vi "BMark_User Visible Strings.vi"() -> ()   [LabVIEW 2013]
panel:
  in  "Switch App Instance":string="LabVIEW cannot locate the specified application instance. "
  in  "Cannot Highlight (missing)":string="The reference for this label is no longer valid."
  in  "Cannot Highlight (lock)":string="Front panel objects in a locked VI (or a VI without a block diagram) cannot be highlighted."
  in  "Cannot Highlight (VI moved)":string="The VI you are trying to open was moved, deleted, or renamed."
  in  "Cannot Highlight (pwd)":string="Labels in a password-protected VI cannot be highlighted if the password is not in the cache."
  in  "Cannot Highlight (run)":string="You cannot highlight labels in a running VI (or a subVI of a running VI)."
  in  "Populating list":string="Populating list... Please wait"
  in  "More Information":string="More Information"
  in  "no bookmarks found":string="No bookmarks found."
  in  "Bookmarks":string="Bookmarks"
  in  "VIs":string="VIs"
  in  "Main application instance":string="Main Application Instance"
  in  "unknown message error":string="The invalid message string \"%s\" was received in the Message Handling Loop."
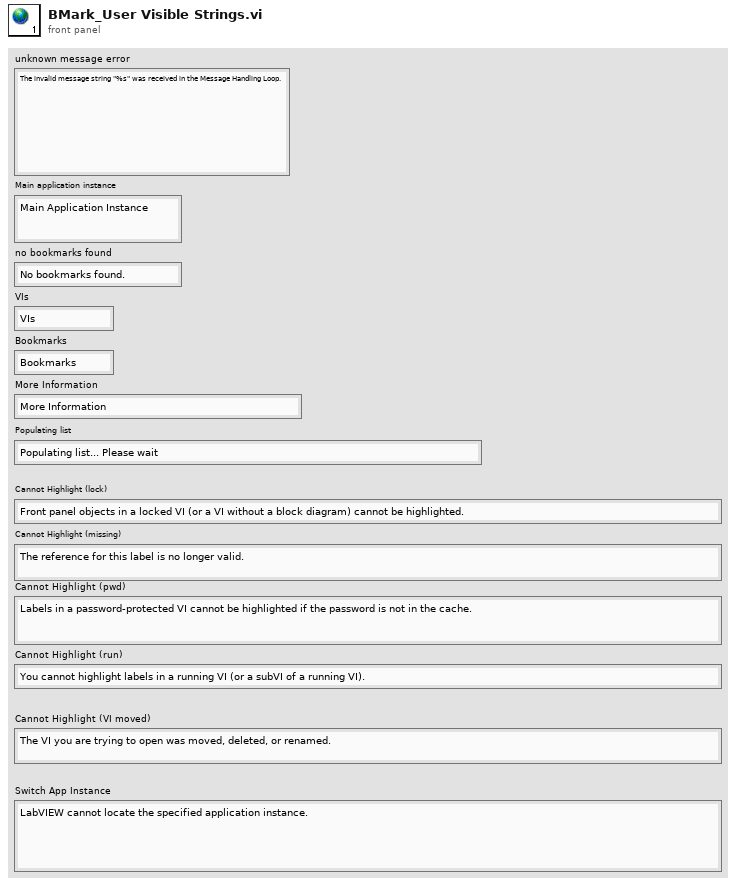
[diagram p1: front panel]
diagram:
